vi "runscenario process Conditions - Add Condition.vi"(6 "Condition Count (0)":i32, 10 "Condition":T1, 11 "Conditions (empty)":T3) -> (3 "Conditions":T3)   [LabVIEW 2011]
uses:
  Addons/internet/utils/keyedarr.llb/Keyed Array.ctl
  server/database/Scenarios/Conditions/Condition Record.ctl
  server/database/Scenarios/Conditions/Condition Operators.ctl
  server/DataFinder/DataFinder Comparisons.ctl
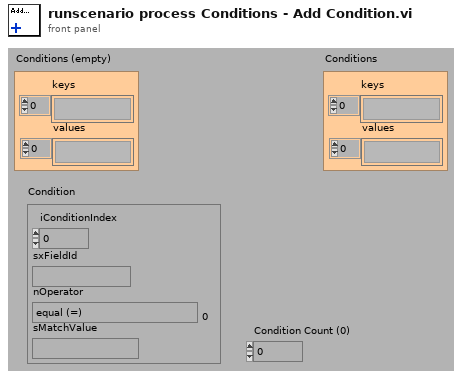
[diagram p1: front panel]
types:
  T1 = typedef "Condition Record.ctl" = cluster{"iConditionIndex":i32, "sxFieldId":string, "nOperator":T2, "sMatchValue":string}
  T2 = typedef "Condition Operators.ctl" = enum16{"equal (=)", "not equal (\\u2260)", "less than (<)", "less than or equal (\\u2264)", "greater than (>)", "greater than or equal (\\u2265)", "contains", "does not contain"}
  T3 = typedef "Keyed Array.ctl" = cluster{"keys":string[], "values":string[]}
  T4 = typedef "DataFinder Comparisons.ctl" = enum16{"=", "<>", "<", "<=", ">", ">="}
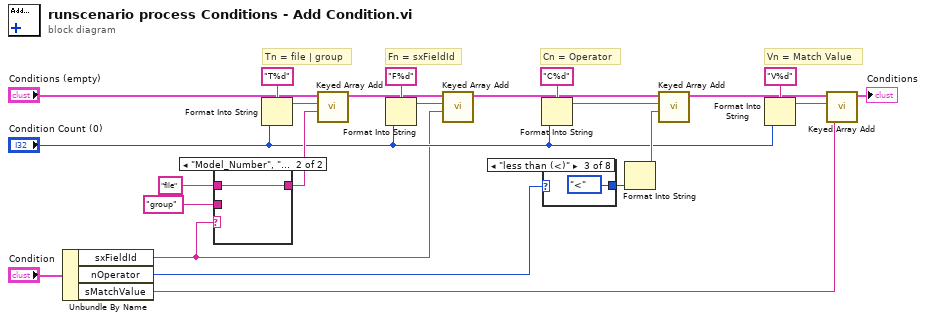
[diagram p0: block diagram]
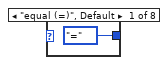
[diagram p3: hidden frame]
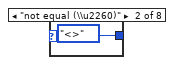
[diagram p4: hidden frame]
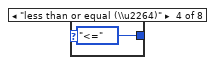
[diagram p5: hidden frame]
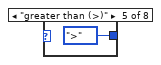
[diagram p6: hidden frame]
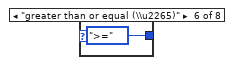
[diagram p7: hidden frame]
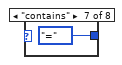
[diagram p8: hidden frame]
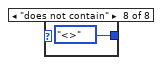
[diagram p9: hidden frame]
diagram:
  # "Tn = file | group"
  # "Vn = Match Value"
  # "Cn = Operator"
  # "Fn = sxFieldId"
  n1 = Unbundle By Name("Condition") -> ("sxFieldId"=w3:string, "nOperator"=w2:T2, "sMatchValue"=w1:string)
  n2 = case shown="\"Model_Number\", \"Serial_Number\", \"Test_Type\"" w3 {
    tunnel: [w24 w25] -> w11
    tunnel: "file" ("key") -> [_ w25]
    tunnel: "group" ("key") -> [w24 _]
    frame "Default", Default {
    }
    frame "Model_Number", "Serial_Number", "Test_Type" {
    }
  }
  n3 = Format Into String(format string="T%d", "Condition Count (0)") -> (resulting string=w12:string)  [unwired: 2 in, 1 out]
  n4 = call "Keyed Array Add.vi"("value"=w11, "key"=w12, "array in"="Conditions (empty)") -> ("array out"=w8:T3)  [unwired: 1 in, 3 out]
  n5 = Format Into String(format string="F%d", "Condition Count (0)") -> (resulting string=w18:string)  [unwired: 2 in, 1 out]
  n6 = call "Keyed Array Add.vi"("value"=w3, "key"=w18, "array in"=w8) -> ("array out"=w19:T3)  [unwired: 1 in, 3 out]
  n7 = Format Into String(format string="C%d", "Condition Count (0)") -> (resulting string=w17:string)  [unwired: 2 in, 1 out]
  n8 = case shown="\"less than (<)\"" w2 {
    tunnel: [DataFinder_Comparisons."=" ("DataFinder Comparisons") DataFinder_Comparisons."<>" ("DataFinder Comparisons") DataFinder_Comparisons."<" ("DataFinder Comparisons") DataFinder_Comparisons."<=" ("DataFinder Comparisons") DataFinder_Comparisons.">" ("DataFinder Comparisons") DataFinder_Comparisons.">=" ("DataFinder Comparisons") DataFinder_Comparisons."=" ("DataFinder Comparisons") DataFinder_Comparisons."<>" ("DataFinder Comparisons")] -> w15
    frame "equal (=)", Default {
    }
    frame "not equal (\\u2260)" {
    }
    frame "less than (<)" {
    }
    frame "less than or equal (\\u2264)" {
    }
    frame "greater than (>)" {
    }
    frame "greater than or equal (\\u2265)" {
    }
    frame "contains" {
    }
    frame "does not contain" {
    }
  }
  n9 = Format Into String(w15) -> (resulting string=w14:string)  [unwired: 3 in, 1 out]
  n10 = call "Keyed Array Add.vi"("value"=w14, "key"=w17, "array in"=w19) -> ("array out"=w20:T3)  [unwired: 1 in, 3 out]
  n11 = Format Into String(format string="V%d", "Condition Count (0)") -> (resulting string=w16:string)  [unwired: 2 in, 1 out]
  n12 = call "Keyed Array Add.vi"("value"=w1, "key"=w16, "array in"=w20) -> ("array out"=→"Conditions":T3)  [unwired: 1 in, 3 out]
